vi "Digital Out Write.vi"(8 "error in (no error)":errorcluster, 10 "Numeric Control":u64, 11 "CAP-USB-1 in":refnum<class "CAP-USB-1.lvclass">) -> (0 "error out":errorcluster, 3 "CAP-USB-1 out":refnum<class "CAP-USB-1.lvclass">)   [LabVIEW 2014, in "CAP-USB-1.lvlib" / "CAP-USB-1.lvclass"]
doc: "Escribe las salidas del dispositivo especificadas"
uses:
  CAP-USB-1.lvclass
  CAP-USB-1.lvclass/CAP-USB-1.ctl
  API/CAP-USB/CAP-USB.lvlib
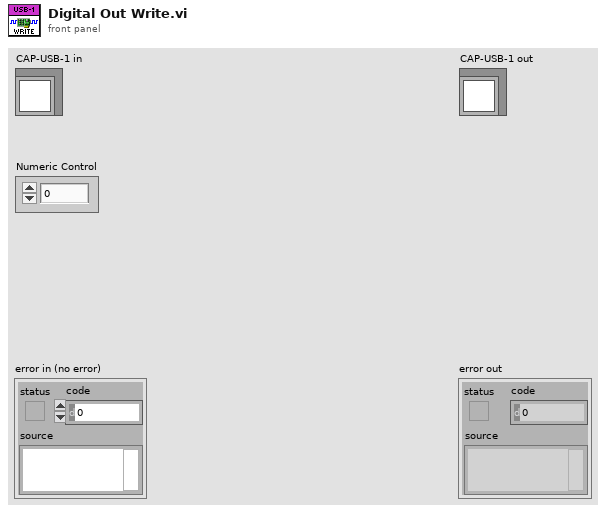
[diagram p1: front panel]
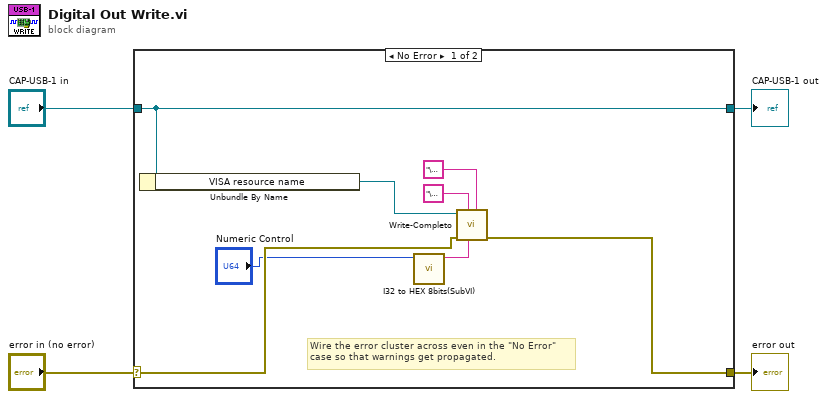
[diagram p0: block diagram]
diagram:
  n1 = case shown="No Error" "error in (no error)" {
    selector: "error in (no error)" -> [w7 w14]
    tunnel: [w6 w14] -> w3
    tunnel: [w9 w13] -> w1
    tunnel: "CAP-USB-1 in" -> [w9 w13]
    frame No Error {
      # "Wire the error cluster across even in the \"No Error\"\ncase so that warnings get propagated."
      n2 = Unbundle By Name(w9) -> ("VISA resource name"=w8:refnum<visa-resource-name>)
      n3 = call "I32 to HEX 8bits(SubVI).vi"("IN U64"="Numeric Control") -> ("OUT HEX 8BITS"=w10:string)  [unwired: 10 in]
      n4 = call "Write-Completo.vi"("Low Byte"="\u0001" ("Hi Byte"), "Dato 8 bits"=w10, "Hi Byte"="\u0003", "error in (no error)"=w7, "VISA resource name"=w8) -> ("error out"=w6:errorcluster)  [unwired: 5 in, 1 out]
    }
    frame Error {
    }
  }
  "error out" <- w3
  "CAP-USB-1 out" <- w1
